vi "get all filenames in cache.vi"(11 "class cache data":T1) -> (3 "Array":string[](array[string]))   [LabVIEW 2013, in "PL_class cache.lvlib"]
uses:
  PL_class cache.lvlib
  cached class information.ctl
  target class metadata.ctl
  class metadata.ctl
  <vilib>/NI/Tag Bus Module Framework/root configuration/Target Types.ctl
  <vilib>/NI/Tag Bus Module Framework/root configuration/TBM configuration.lvclass
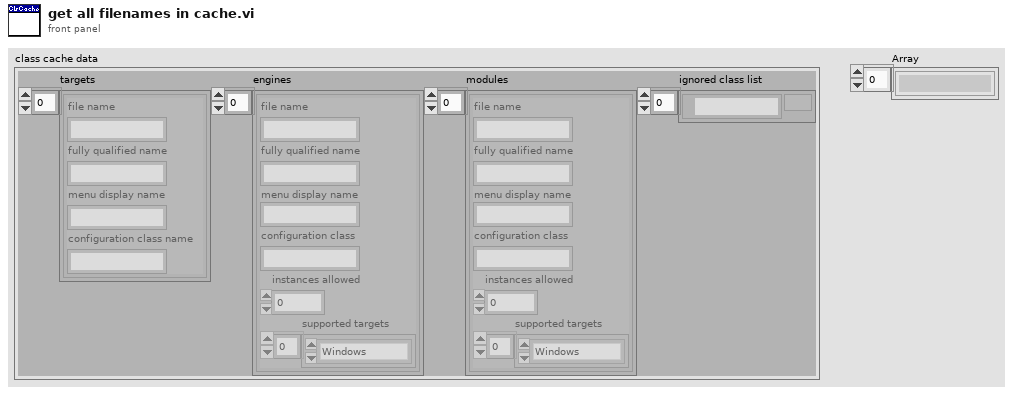
[diagram p1: front panel]
types:
  T1 = typedef "PL_class cache.lvlib/cached class information.ctl" = cluster{"targets":T2[], "engines":T3[], "modules":T3[], "ignored class list":path[]}
  T2 = typedef "PL_class cache.lvlib/target class metadata.ctl" = cluster{"file name":string, "fully qualified name":string, "menu display name":string, "configuration class name":string}
  T3 = typedef "PL_class cache.lvlib/class metadata.ctl" = cluster{"file name":string, "fully qualified name":string, "menu display name":string, "configuration class":string, "instances allowed":i32, "supported targets":T4[]}
  T4 = typedef "TBM configuration.lvclass/Target Types.ctl" = enum16{"Windows", "Mac", "Linux", "Linux RT ARM", "VxWorks", "Pharlap", "Other", "Linux RT x64"}
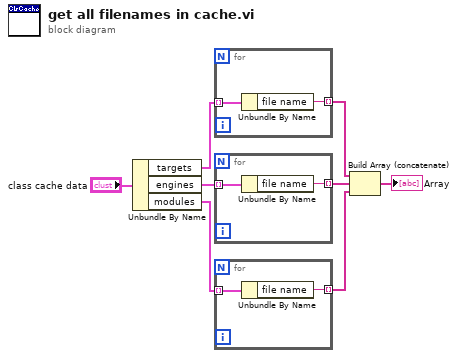
[diagram p0: block diagram]
diagram:
  n1 = Unbundle By Name("class cache data") -> ("targets"=w2:T2[], "engines"=w4:T3[], "modules"=w3:T3[])
  n2 = for {
    tunnel: w2 -> [w10] mode=indexing
    tunnel: [w9] -> w7 mode=indexing
    n3 = Unbundle By Name(w10) -> ("file name"=w9:string)
  }
  n4 = for {
    tunnel: w4 -> [w12] mode=indexing
    tunnel: [w11] -> w6 mode=indexing
    n5 = Unbundle By Name(w12) -> ("file name"=w11:string)
  }
  n6 = for {
    tunnel: w3 -> [w14] mode=indexing
    tunnel: [w13] -> w5 mode=indexing
    n7 = Unbundle By Name(w14) -> ("file name"=w13:string)
  }
  n8 = Build Array (concatenate)(w7, w6, w5) -> (→"Array":string[])
